vi "Get Temperature Coefficient.vi"(8 "error in (no error)":errorcluster, 10 "Channel":T1, 11 "EPU452 in":refnum<class "EPU452.lvclass">) -> (0 "error out":errorcluster, 1 "Temperature Coefficient":dbl, 2 "Response":string, 3 "EPU452 out":refnum<class "EPU452.lvclass">)   [LabVIEW 2018, in "EPU452.lvclass"]
uses:
  EPU452.lvclass
  Controls/Channels.ctl
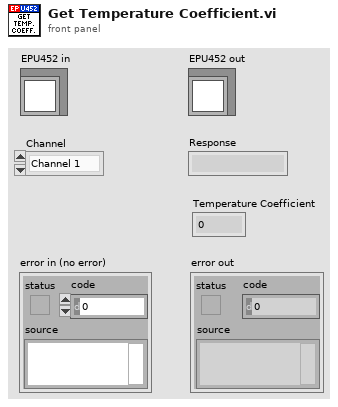
[diagram p1: front panel]
types:
  T1 = typedef "EPU452.lvclass/Channels.ctl" = enum16{"Channel 1", "Channel 2", "Channel 3", "Channel 4"}
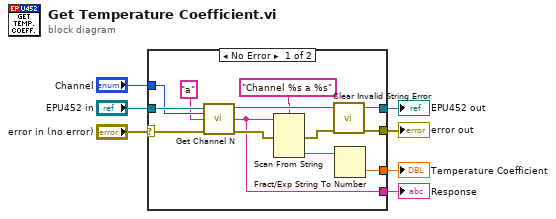
[diagram p0: block diagram]
diagram:
  n1 = case shown="No Error" "error in (no error)" {
    selector: "error in (no error)" -> [w18 w22]
    tunnel: [w11 w22] -> w6
    tunnel: [w10 w21] -> w4
    tunnel: "EPU452 in" -> [w20 w21]
    tunnel: "Channel" -> [w19 _]
    tunnel: [w9 _] -> w2
    tunnel: [w8 _] -> w1
    frame No Error {
      n2 = call "Get Channel N.vi"("EPU452 in"=w20, "Channel"=w19, "Function"="a", "error in (no error)"=w18) -> ("EPU452 out"=w15:refnum<class "EPU452.lvclass">, "Response"=w8:string, "error out"=w16:errorcluster)  [unwired: 9 in]
      n3 = Scan From String(format string="Channel %s a %s", input string=w8, error in=w16) -> (error out=w13:errorcluster, output 2=w12:string)  [unwired: 4 in, 2 out]
      n4 = call "Clear Invalid String Error.vi"("error in (no error)"=w13, "EPU452 in"=w15) -> ("error out"=w11:errorcluster, "EPU452 out"=w10:refnum<class "EPU452.lvclass">)  [unwired: 8 in]
      n5 = Fract/Exp String To Number(string=w12) -> (number=w9:dbl)  [unwired: 3 in, 1 out]
    }
    frame Error {
    }
  }
  "error out" <- w6
  "EPU452 out" <- w4
  "Temperature Coefficient" <- w2
  "Response" <- w1
